vi "file_indexing.vi"(8 "Sigfig":dbl, 10 "path":path) -> (1 "output cluster":T1, 3 "stripped path":path)   [LabVIEW 2013]
uses:
  <vilib>/Utility/file.llb/Read From Spreadsheet File (DBL).vi
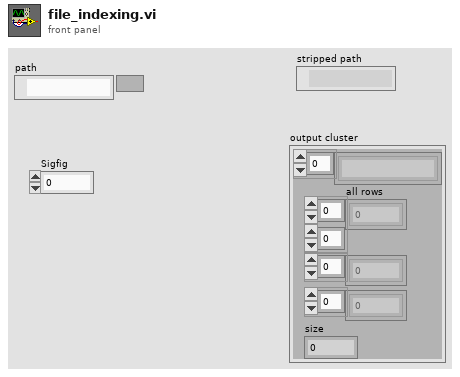
[diagram p1: front panel]
types:
  T1 = cluster{string[], "all rows":dbl[][], i32[], i32[], "size":i64}
  T2 = cluster{string[], "all rows":dbl[][], "x/y":dbl[], "x/y":dbl[], i32}
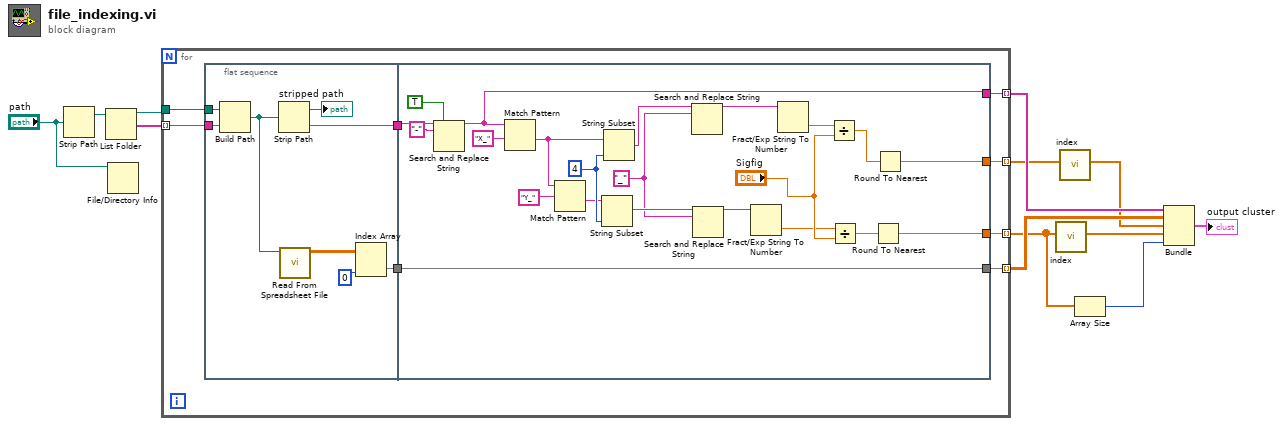
[diagram p0: block diagram]
diagram:
  n1 = Strip Path(path="path") -> (stripped path=w7:path)  [unwired: 1 out]
  n2 = List Folder(path=w7) -> (path out=w12:path, filenames=w5:string[])  [unwired: 3 in, 2 out]
  n3 = File/Directory Info(path="path") -> ()  [unwired: 1 in, 7 out]
  n4 = for {
    tunnel: w5 -> [w20] mode=indexing
    tunnel: w12 -> [w19]
    tunnel: [w17] -> w4 mode=indexing
    tunnel: [w16] -> w8 mode=indexing
    tunnel: [w15] -> w10 mode=indexing
    tunnel: [w14] -> w11 mode=indexing
    n5 = flat-sequence {
      tunnel: w20 -> [w28]
      tunnel: w19 -> [w24]
      tunnel: [w27] -> w18
      tunnel: [w25] -> w13
      tunnel: w18 -> [w39]
      tunnel: [w35] -> w16
      tunnel: [w34] -> w17
      tunnel: [w38] -> w15
      tunnel: [w43] -> w14
      tunnel: w13 -> [w43]
      frame #0 {
        n6 = Build Path(base path=w24, name or relative path=w28) -> (appended path=w23:path)
        n7 = Strip Path(path=w23) -> (stripped path=→"stripped path":path, name=w27:string)
        n8 = call-poly <vilib>:"Read From Spreadsheet File.vi"("file path (dialog if empty)"=w23) -> ("all rows"=w22:dbl[][])  [unwired: 6 in, 4 out]
        n9 = Index Array(array=w22, index (col)=0 ("disabled index (col)")) -> (element=w25:dbl[])  [unwired: 1 in]
      }
      frame #1 {
        w44 = "_" ("search string")
        w49 = 4 ("length (rest)")
        n10 = Search and Replace String(replace all?=TRUE ("replace all? (F)"), input string=w39, search string="-") -> (result string=w38:string)  [unwired: 5 in, 3 out]
        n11 = Match Pattern(string=w38, regular expression="X_") -> (after substring=w42:string)  [unwired: 1 in, 3 out]
        n12 = Match Pattern(string=w42, regular expression="Y_") -> (after substring=w47:string)  [unwired: 1 in, 3 out]
        n13 = String Subset(string=w47, length (rest)=w49) -> (substring=w46:string)  [unwired: 1 in]
        n14 = String Subset(string=w42, length (rest)=w49) -> (substring=w45:string)  [unwired: 1 in]
        n15 = Search and Replace String(input string=w45, search string=w44) -> (result string=w41:string)  [unwired: 6 in, 3 out]
        n16 = Search and Replace String(input string=w46, search string=w44) -> (result string=w40:string)  [unwired: 6 in, 3 out]
        n17 = Fract/Exp String To Number(string=w40) -> (number=w31:dbl)  [unwired: 3 in, 1 out]
        n18 = Fract/Exp String To Number(string=w41) -> (number=w32:dbl)  [unwired: 3 in, 1 out]
        n19 = Divide(x=w32, y="Sigfig") -> (x/y=w29:dbl)
        n20 = Divide(x=w31, y="Sigfig") -> (x/y=w30:dbl)
        n21 = Round To Nearest(number=w30) -> (nearest integer value=w34:dbl)
        n22 = Round To Nearest(number=w29) -> (nearest integer value=w35:dbl)
      }
    }
  }
  n23 = call "index.vi"("Array"=w4) -> ("x/y"=w1:dbl[])  [unwired: 10 in]
  n24 = call "index.vi"("Array"=w8) -> ("x/y"=w2:dbl[])  [unwired: 10 in]
  n25 = Array Size(array=w4) -> (size(s)=w3:i32)
  n26 = Bundle(w10, "all rows"=w11, "x/y"=w2, "x/y"=w1, w3) -> (→"output cluster":T2)  [unwired: 1 in]
